vi "Destroy Class ObjectData DVR.vi"(8 "error in (no error)":errorcluster, 11 "DbgTimers in":refnum<class "DbgTimers.lvclass">) -> (0 "error out":errorcluster, 3 "DbgTimers out":refnum<class "DbgTimers.lvclass">)   [LabVIEW 2017, in "DbgTimers.lvclass"]
doc: "Developed by Kevin Thompson\nkevin@thompsonengineering.net\n\nCopyright 2018-2020\nThompson Engineering, LLC"
uses:
  DbgTimers.lvclass
  DbgTimers.lvclass/DbgTimers.ctl
panel:
  out "ObjData AsVariant":variant
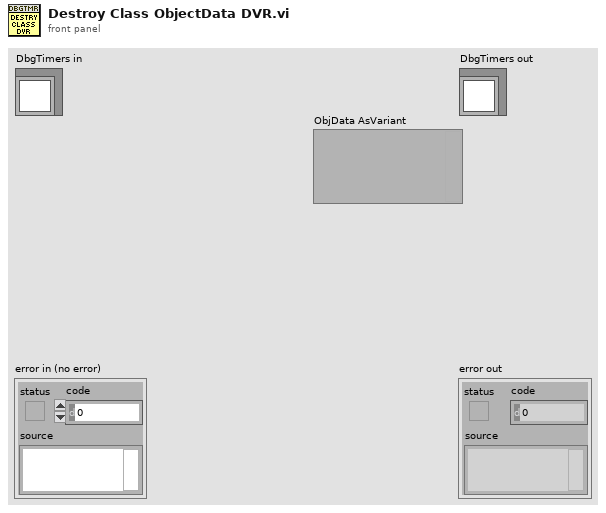
[diagram p1: front panel]
types:
  T1 = typedef "DbgTimers.lvclass/ObjData--cluster.ctl" = cluster{"Settings":T2, "ReadData-placeholder":T3, "Timers":T4, "Enable msTick Logging":bool, "LogFile_msTickTimer":path}
  T2 = typedef "DbgTimers.lvclass/Settings--cluster.ctl" = cluster{"Simulation":bool, "DbgTimer LogFolder":path}
  T3 = typedef "DbgTimers.lvclass/Read Data--cluster.ctl" = cluster{"Data":dbl}
  T4 = typedef "DbgTimers.lvclass/Timers--cluster.ctl" = cluster{"ms tick timers":T5[]}
  T5 = typedef "DbgTimers.lvclass/Millisecond Tick Timer--cluster.ctl" = cluster{"startTick":u32, "currentTick":u32, "elapsedTicks":u32, "totalElapsedTicks":u32}
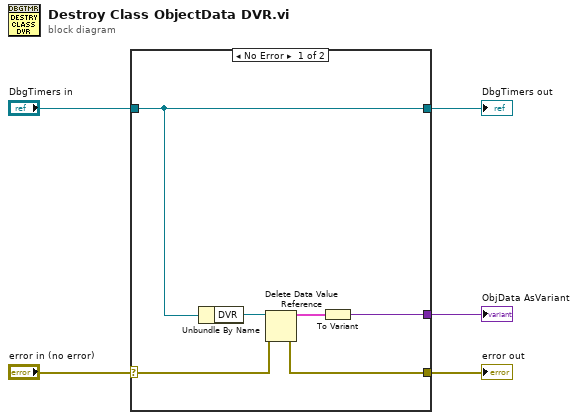
[diagram p0: block diagram]
diagram:
  n1 = case shown="No Error" "error in (no error)" {
    selector: "error in (no error)" -> [w11 w13]
    tunnel: [w10 w13] -> w4
    tunnel: [w8 w12] -> w2
    tunnel: "DbgTimers in" -> [w8 w12]
    tunnel: [w6 _] -> w1
    frame No Error {
      n2 = Unbundle By Name(w8) -> ("DVR"=w9:refnum<data-value>)
      n3 = Delete Data Value Reference(data value reference=w9, error in=w11) -> (data value=w7:T1, error out=w10:errorcluster)
      n4 = To Variant(anything=w7) -> (Variant=w6:variant)
    }
    frame Error {
    }
  }
  "error out" <- w4
  "DbgTimers out" <- w2
  "ObjData AsVariant" <- w1
